vi "Shortcuts.vi"() -> (3 "LINX Shortcuts":T1[](array[typedef]))   [LabVIEW 2019, in "LINX.lvlib" / "LINX.lvclass"]
uses:
  LINX.lvclass
  LINX Shortcut.ctl
  LINX Channel Type.ctl
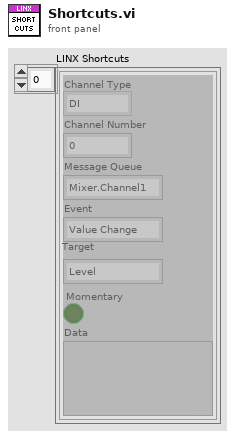
[diagram p1: front panel]
types:
  T1 = typedef "LINX.lvlib/LINX.lvclass/LINX Shortcut.ctl" = cluster{"Channel Type":T2, "Channel Number":u8, "Message Queue":string, "Event":string, "Target":string, "Momentary":bool, "Data":variant}
  T2 = typedef "LINX.lvlib/LINX.lvclass/LINX Channel Type.ctl" = enum16{"DI", "AI"}
  T3 = typedef "LINX.lvlib/LINX.lvclass/LINX Shortcut.ctl" = cluster{"DAQmx Global Channel":refnum<k21>, "Message Queue":string, "Event":string, "Target":string, "Momentary":bool, "Data":variant}
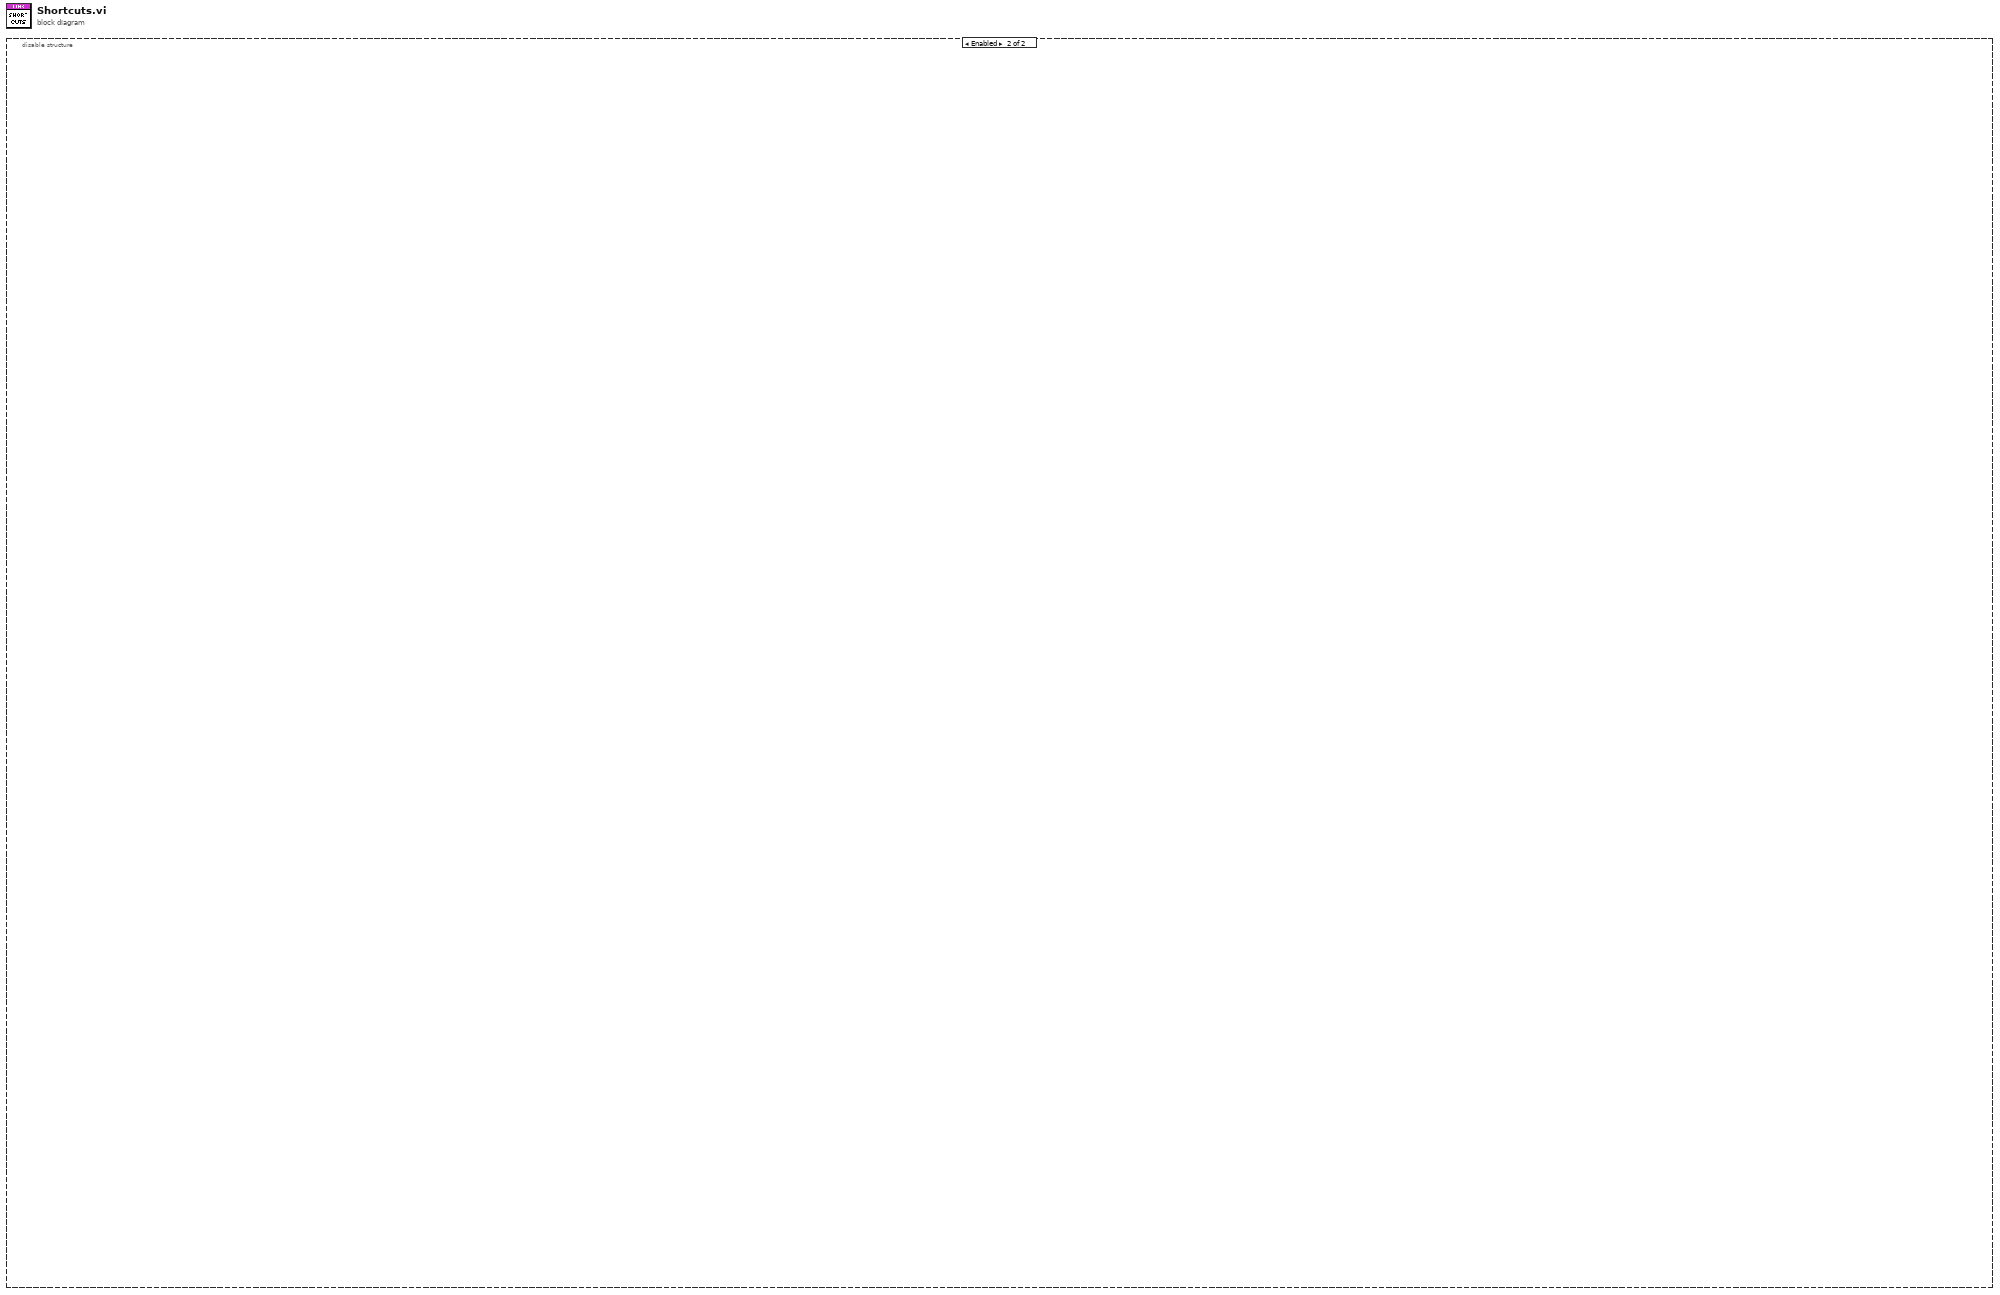
[diagram p0: block diagram]
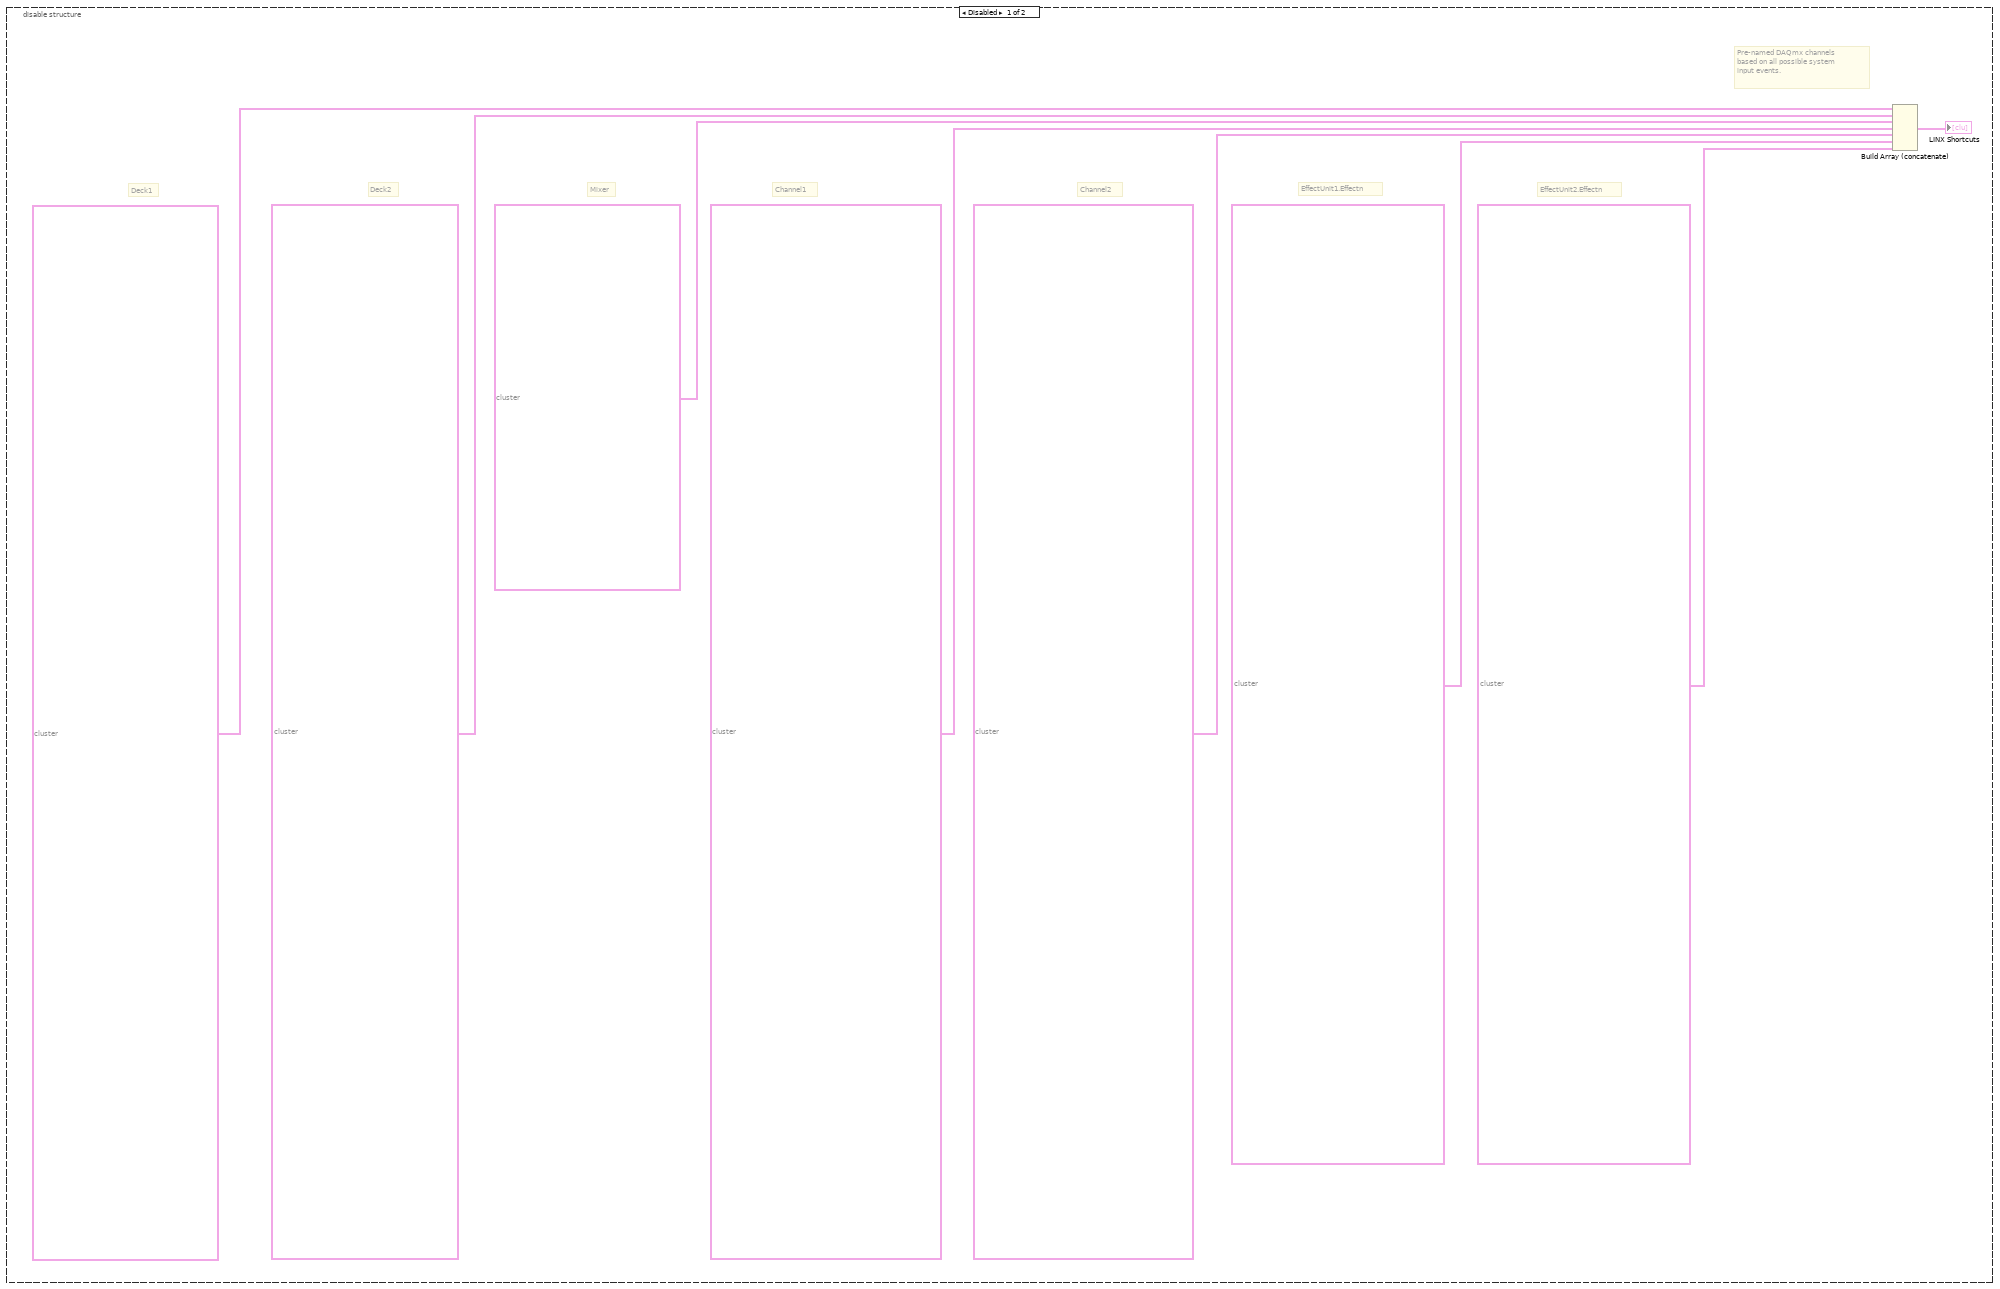
[diagram p2: hidden frame]
diagram:
  n1 = disable-structure shown="Enabled" {
    frame Disabled {
      # "Deck2"
      # "Deck1"
      # "EffectUnit2.Effectn"
      # "EffectUnit1.Effectn"
      # "Channel2"
      # "Channel1"
      # "Mixer"
      # "Pre-named DAQmx channels based on all possible system input events."
      n2 = Build Array (concatenate)(T3[] [{"DAQmx Global Channel"="Deck1_Play", "Message Queue"="Deck1", "Event"="Toggle", "Target"="Play", "Momentary"=FALSE, "Data"=variant}, {"DAQmx Global Channel"="Deck1_Brake", "Message Queue"="Deck1", "Event"="Toggle", "Target"="Brake", "Momentary"=FALSE, "Data"=variant}, {"DAQmx Global Channel"="Deck1_Backspin", "Message Queue"="Deck1", "Event"="Toggle", "Target"="Backspin", "Momentary"=FALSE, "Data"=variant}, {"DAQmx Global Channel"="Deck1_Reverse", "Message Queue"="Deck1", "Event"="Toggle", "Target"="Reverse", "Momentary"=FALSE, "Data"=variant}, {"DAQmx Global Channel"="Deck1_Cue1", "Message Queue"="Deck1", "Event"="Value Change", "Target"="Cue1", "Momentary"=FALSE, "Data"=variant}, {"DAQmx Global Channel"="Deck1_Cue2", "Message Queue"="Deck1", "Event"="Value Change", "Target"="Cue2", "Momentary"=FALSE, "Data"=variant}, {"DAQmx Global Channel"="Deck1_Cue3", "Message Queue"="Deck1", "Event"="Value Change", "Target"="Cue3", "Momentary"=FALSE, "Data"=variant}, {"DAQmx Global Channel"="Deck1_PitchBendDown", "Message Queue"="Deck1", "Event"="Value Change", "Target"="PitchBendDown", "Momentary"=TRUE, "Data"=variant}, {"DAQmx Global Channel"="Deck1_PitchBendUp", "Message Queue"="Deck1", "Event"="Value Change", "Target"="PitchBendUp", "Momentary"=TRUE, "Data"=variant}, {"DAQmx Global Channel"="Deck1_Pitch", "Message Queue"="Deck1", "Event"="Value Change", "Target"="Pitch", "Momentary"=FALSE, "Data"=variant}], T3[] [{"DAQmx Global Channel"="Deck2_Play", "Message Queue"="Deck2", "Event"="Toggle", "Target"="Play", "Momentary"=FALSE, "Data"=variant}, {"DAQmx Global Channel"="Deck2_Brake", "Message Queue"="Deck2", "Event"="Toggle", "Target"="Brake", "Momentary"=FALSE, "Data"=variant}, {"DAQmx Global Channel"="Deck2_Backspin", "Message Queue"="Deck2", "Event"="Toggle", "Target"="Backspin", "Momentary"=FALSE, "Data"=variant}, {"DAQmx Global Channel"="Deck2_Reverse", "Message Queue"="Deck2", "Event"="Toggle", "Target"="Reverse", "Momentary"=FALSE, "Data"=variant}, {"DAQmx Global Channel"="Deck2_Cue1", "Message Queue"="Deck2", "Event"="Value Change", "Target"="Cue1", "Momentary"=FALSE, "Data"=variant}, {"DAQmx Global Channel"="Deck2_Cue2", "Message Queue"="Deck2", "Event"="Value Change", "Target"="Cue2", "Momentary"=FALSE, "Data"=variant}, {"DAQmx Global Channel"="Deck2_Cue3", "Message Queue"="Deck2", "Event"="Value Change", "Target"="Cue3", "Momentary"=FALSE, "Data"=variant}, {"DAQmx Global Channel"="Deck2_PitchBendDown", "Message Queue"="Deck2", "Event"="Value Change", "Target"="PitchBendDown", "Momentary"=TRUE, "Data"=variant}, {"DAQmx Global Channel"="Deck2_PitchBendUp", "Message Queue"="Deck2", "Event"="Value Change", "Target"="PitchBendUp", "Momentary"=TRUE, "Data"=variant}, {"DAQmx Global Channel"="Deck2_Pitch", "Message Queue"="Deck2", "Event"="Value Change", "Target"="Pitch", "Momentary"=FALSE, "Data"=variant}], T3[] [{"DAQmx Global Channel"="Mixer_Master", "Message Queue"="Mixer", "Event"="Value Change", "Target"="Master", "Momentary"=FALSE, "Data"=variant}, {"DAQmx Global Channel"="Mixer_Headphones", "Message Queue"="Mixer", "Event"="Value Change", "Target"="Headphones", "Momentary"=FALSE, "Data"=variant}, {"DAQmx Global Channel"="Mixer_Crossfader", "Message Queue"="Mixer", "Event"="Value Change", "Target"="Crossfader", "Momentary"=FALSE, "Data"=variant}], T3[] [{"DAQmx Global Channel"="Channel1_Gain", "Message Queue"="Channel1", "Event"="Value Change", "Target"="Gain", "Momentary"=FALSE, "Data"=variant}, {"DAQmx Global Channel"="Channel1_Level", "Message Queue"="Channel1", "Event"="Value Change", "Target"="Level", "Momentary"=FALSE, "Data"=variant}, {"DAQmx Global Channel"="Channel1_EQHigh", "Message Queue"="Channel1", "Event"="Value Change", "Target"="EQHigh", "Momentary"=FALSE, "Data"=variant}, {"DAQmx Global Channel"="Channel1_EQMid", "Message Queue"="Channel1", "Event"="Value Change", "Target"="EQMid", "Momentary"=FALSE, "Data"=variant}, {"DAQmx Global Channel"="Channel1_EQLow", "Message Queue"="Channel1", "Event"="Value Change", "Target"="EQLow", "Momentary"=FALSE, "Data"=variant}, {"DAQmx Global Channel"="Channel1_EQFilter", "Message Queue"="Channel1", "Event"="Value Change", "Target"="EQFilter", "Momentary"=FALSE, "Data"=variant}, {"DAQmx Global Channel"="Channel1_EQHighKill", "Message Queue"="Channel1", "Event"="Toggle", "Target"="EQHighKill", "Momentary"=FALSE, "Data"=variant}, {"DAQmx Global Channel"="Channel1_EQMidKill", "Message Queue"="Channel1", "Event"="Toggle", "Target"="EQMidKill", "Momentary"=FALSE, "Data"=variant}, {"DAQmx Global Channel"="Channel1_EQLowKill", "Message Queue"="Channel1", "Event"="Toggle", "Target"="EQLowKill", "Momentary"=FALSE, "Data"=variant}, {"DAQmx Global Channel"="Channel1_HeadphoneOutput", "Message Queue"="Channel1", "Event"="Toggle", "Target"="HeadphoneOutput", "Momentary"=FALSE, "Data"=variant}], T3[] [{"DAQmx Global Channel"="Channel2_Gain", "Message Queue"="Channel2", "Event"="Value Change", "Target"="Gain", "Momentary"=FALSE, "Data"=variant}, {"DAQmx Global Channel"="Channel2_Level", "Message Queue"="Channel2", "Event"="Value Change", "Target"="Level", "Momentary"=FALSE, "Data"=variant}, {"DAQmx Global Channel"="Channel2_EQHigh", "Message Queue"="Channel2", "Event"="Value Change", "Target"="EQHigh", "Momentary"=FALSE, "Data"=variant}, {"DAQmx Global Channel"="Channel2_EQMid", "Message Queue"="Channel2", "Event"="Value Change", "Target"="EQMid", "Momentary"=FALSE, "Data"=variant}, {"DAQmx Global Channel"="Channel2_EQLow", "Message Queue"="Channel2", "Event"="Value Change", "Target"="EQLow", "Momentary"=FALSE, "Data"=variant}, {"DAQmx Global Channel"="Channel2_EQFilter", "Message Queue"="Channel2", "Event"="Value Change", "Target"="EQFilter", "Momentary"=FALSE, "Data"=variant}, {"DAQmx Global Channel"="Channel2_EQHighKill", "Message Queue"="Channel2", "Event"="Toggle", "Target"="EQHighKill", "Momentary"=FALSE, "Data"=variant}, {"DAQmx Global Channel"="Channel2_EQMidKill", "Message Queue"="Channel2", "Event"="Toggle", "Target"="EQMidKill", "Momentary"=FALSE, "Data"=variant}, {"DAQmx Global Channel"="Channel2_EQLowKill", "Message Queue"="Channel2", "Event"="Toggle", "Target"="EQLowKill", "Momentary"=FALSE, "Data"=variant}, {"DAQmx Global Channel"="Channel2_HeadphoneOutput", "Message Queue"="Channel2", "Event"="Toggle", "Target"="HeadphoneOutput", "Momentary"=FALSE, "Data"=variant}], T3[] [{"DAQmx Global Channel"="EffectUnit1_Effect1_Value1", "Message Queue"="EffectUnit1.Effect1", "Event"="Value Change", "Target"="Value1", "Momentary"=FALSE, "Data"=variant}, {"DAQmx Global Channel"="EffectUnit1_Effect1_Value2", "Message Queue"="EffectUnit1.Effect1", "Event"="Value Change", "Target"="Value2", "Momentary"=FALSE, "Data"=variant}, {"DAQmx Global Channel"="EffectUnit1_Effect1_Enable", "Message Queue"="EffectUnit1.Effect1", "Event"="Toggle", "Target"="Enable", "Momentary"=FALSE, "Data"=variant}, {"DAQmx Global Channel"="EffectUnit1_Effect2_Value1", "Message Queue"="EffectUnit1.Effect2", "Event"="Value Change", "Target"="Value1", "Momentary"=FALSE, "Data"=variant}, {"DAQmx Global Channel"="EffectUnit1_Effect2_Value2", "Message Queue"="EffectUnit1.Effect2", "Event"="Value Change", "Target"="Value2", "Momentary"=FALSE, "Data"=variant}, {"DAQmx Global Channel"="EffectUnit1_Effect2_Enable", "Message Queue"="EffectUnit1.Effect2", "Event"="Toggle", "Target"="Enable", "Momentary"=FALSE, "Data"=variant}, {"DAQmx Global Channel"="EffectUnit1_Effect3_Value1", "Message Queue"="EffectUnit1.Effect3", "Event"="Value Change", "Target"="Value1", "Momentary"=FALSE, "Data"=variant}, {"DAQmx Global Channel"="EffectUnit1_Effect3_Value2", "Message Queue"="EffectUnit1.Effect3", "Event"="Value Change", "Target"="Value2", "Momentary"=FALSE, "Data"=variant}, {"DAQmx Global Channel"="EffectUnit1_Effect3_Enable", "Message Queue"="EffectUnit1.Effect3", "Event"="Toggle", "Target"="Enable", "Momentary"=FALSE, "Data"=variant}], T3[] [{"DAQmx Global Channel"="EffectUnit2_Effect1_Value1", "Message Queue"="EffectUnit2.Effect1", "Event"="Value Change", "Target"="Value1", "Momentary"=FALSE, "Data"=variant}, {"DAQmx Global Channel"="EffectUnit2_Effect1_Value2", "Message Queue"="EffectUnit2.Effect1", "Event"="Value Change", "Target"="Value2", "Momentary"=FALSE, "Data"=variant}, {"DAQmx Global Channel"="EffectUnit2_Effect1_Enable", "Message Queue"="EffectUnit2.Effect1", "Event"="Toggle", "Target"="Enable", "Momentary"=FALSE, "Data"=variant}, {"DAQmx Global Channel"="EffectUnit2_Effect2_Value1", "Message Queue"="EffectUnit2.Effect2", "Event"="Value Change", "Target"="Value1", "Momentary"=FALSE, "Data"=variant}, {"DAQmx Global Channel"="EffectUnit2_Effect2_Value2", "Message Queue"="EffectUnit2.Effect2", "Event"="Value Change", "Target"="Value2", "Momentary"=FALSE, "Data"=variant}, {"DAQmx Global Channel"="EffectUnit2_Effect2_Enable", "Message Queue"="EffectUnit2.Effect2", "Event"="Toggle", "Target"="Enable", "Momentary"=FALSE, "Data"=variant}, {"DAQmx Global Channel"="EffectUnit2_Effect3_Value1", "Message Queue"="EffectUnit2.Effect3", "Event"="Value Change", "Target"="Value1", "Momentary"=FALSE, "Data"=variant}, {"DAQmx Global Channel"="EffectUnit2_Effect3_Value2", "Message Queue"="EffectUnit2.Effect3", "Event"="Value Change", "Target"="Value2", "Momentary"=FALSE, "Data"=variant}, {"DAQmx Global Channel"="EffectUnit2_Effect3_Enable", "Message Queue"="EffectUnit2.Effect3", "Event"="Toggle", "Target"="Enable", "Momentary"=FALSE, "Data"=variant}]) -> (→"LINX Shortcuts":T3[])
    }
    frame Enabled {
    }
  }
